vi "setSetpoint.vi"(8 "error in (no error)":errorcluster, 9 "Force Setpoint":dbl[unit], 10 "ILC in":refnum<class "ILC.lvclass">, 11 "FlowControlActuator in":refnum<class "FlowControlActuator.lvclass">) -> (0 "error out":errorcluster, 2 "ILC out":refnum<class "ILC.lvclass">, 3 "FlowControlActuator out":refnum<class "FlowControlActuator.lvclass">)   [LabVIEW 2015, in "FlowControlActuator.lvclass"]
uses:
  FlowControlActuator.lvclass
  <userlib>/Common/ILC/ILC/ILC.lvclass
  FlowControlActuator.lvclass/FlowControlActuator.ctl
  ActuatorCylinder/IActuatorCylinder/IActuatorCylinder.lvclass
  Calculators/ForceToFlowControlVoltage/ForceToFlowControlVoltage.lvclass
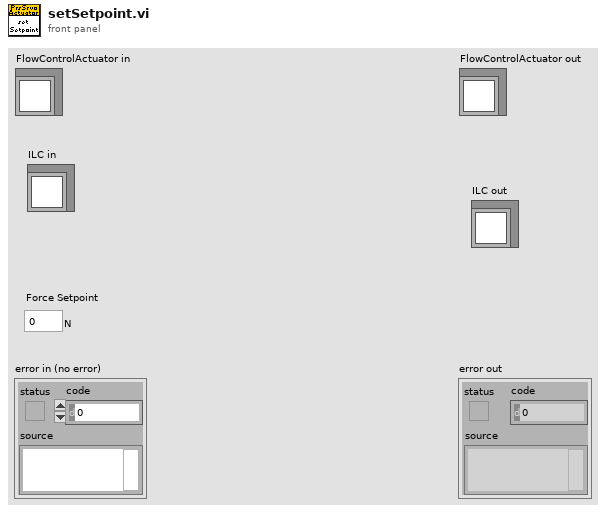
[diagram p1: front panel]
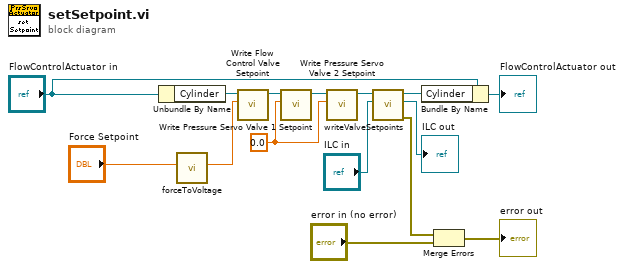
[diagram p0: block diagram]
diagram:
  w3 = dbl[unit] 0.0 ("Flow Control Valve Setpoint")
  n1 = Unbundle By Name("FlowControlActuator in") -> ("Cylinder"=w8:refnum<class "IActuatorCylinder.lvclass">)
  n2 = call "forceToVoltage.vi"("Force"="Force Setpoint") -> ("Voltage"=w1:dbl[unit])  [unwired: 8 in, 2 out]
  n3 = call-dynamic "Write Flow Control Valve Setpoint.vi"("Flow Control Valve Setpoint"=w1, "IActuatorCylinder in"=w8) -> ("IActuatorCylinder out"=w7:refnum<class "IActuatorCylinder.lvclass">)  [unwired: 9 in]
  n4 = call-dynamic "Write Pressure Servo Valve 1 Setpoint.vi"("Pressure Servo Valve 1 Setpoint"=w3, "IActuatorCylinder in"=w7) -> ("IActuatorCylinder out"=w6:refnum<class "IActuatorCylinder.lvclass">)  [unwired: 9 in]
  n5 = call-dynamic "Write Pressure Servo Valve 2 Setpoint.vi"("Pressure Servo Valve 2 Setpoint"=w3, "IActuatorCylinder in"=w6) -> ("IActuatorCylinder out"=w9:refnum<class "IActuatorCylinder.lvclass">)  [unwired: 9 in]
  n6 = call-dynamic "writeValveSetpoints.vi"("ILC in"="ILC in", "IActuatorCylinder in"=w9) -> ("error out"=w13:errorcluster, "ILC out"=→"ILC out":refnum<class "ILC.lvclass">, "IActuatorCylinder out"=w10:refnum<class "IActuatorCylinder.lvclass">)  [unwired: 7 in]
  n7 = Bundle By Name(cluster="FlowControlActuator in", "Cylinder"=w10) -> (→"FlowControlActuator out":refnum<class "FlowControlActuator.lvclass">)
  n8 = Merge Errors(w13, "error in (no error)") -> (→"error out":errorcluster)
